vi "PathPlanner_PathFinder_SetNewPathAvail.vi"(8 "error in (no error)":errorcluster) -> (0 "error out":errorcluster)   [LabVIEW 2019, in "PathPlanner24.lvlib"]
uses:
  PathPlanner_GridPosition_Get.vi
  PathPlanner_GridPosition_New.vi
  PathPlanner_PathFinder_Globals.vi
  PathPlanner24.lvlib
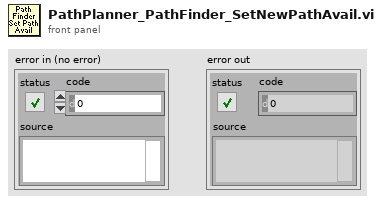
[diagram p1: front panel]
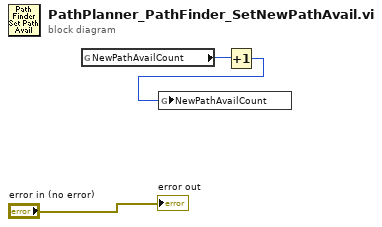
[diagram p0: block diagram]
diagram:
  n1 = global read "PathPlanner_PathFinder_Globals.vi" "NewPathAvailCount"() -> (w3:i32)
  n2 = Increment(x=w3) -> (x+1=w2:i32)
  n3 = global write "PathPlanner_PathFinder_Globals.vi" "NewPathAvailCount"(w2) -> ()
  "error out" <- "error in (no error)"
